vi "Quadratic-Root-Calculation.vi"() -> ()   [LabVIEW 2014]
panel:
  out "x2":dbl
  out "x1":dbl
  in  "c":dbl
  in  "b":dbl
  in  "a":dbl
  # "Quadratic root calculation"
  # "x^2 +"
  # "x +"
  # "Answer"
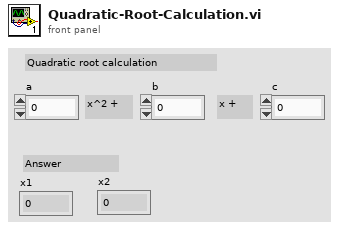
[diagram p1: front panel]
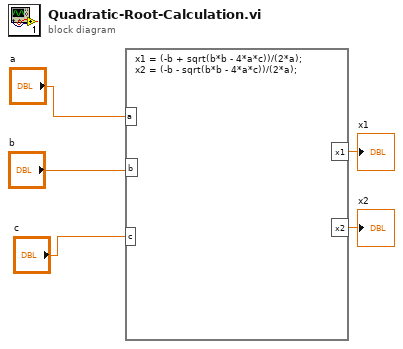
[diagram p0: block diagram]
diagram:
  n1 = formula code="x1 = (-b + sqrt(b*b - 4*a*c))/(2*a);\nx2 = (-b - sqrt(b*b - 4*a*c))/(2*a);"("a"="a", "b"="b", "c"="c") -> ("x1"=→"x1":dbl, "x2"=→"x2":dbl)
